vi "Load XML.vi"(8 "error in (no error)":errorcluster, 11 "path to XML document":path) -> (0 "error out":errorcluster, 3 "Map":map{string, T1}(c390))   [LabVIEW 2025]
uses:
  Controls/bd.ctl
  Classes/Node/Node.lvclass
  Controls/wire.ctl
  Controls/Terminal.ctl
  <vilib>/xml/Load XML File.vi
  <vilib>/xml/NI_XML.lvlib
  <vilib>/httpClient/LabVIEWHTTPClient.lvlib
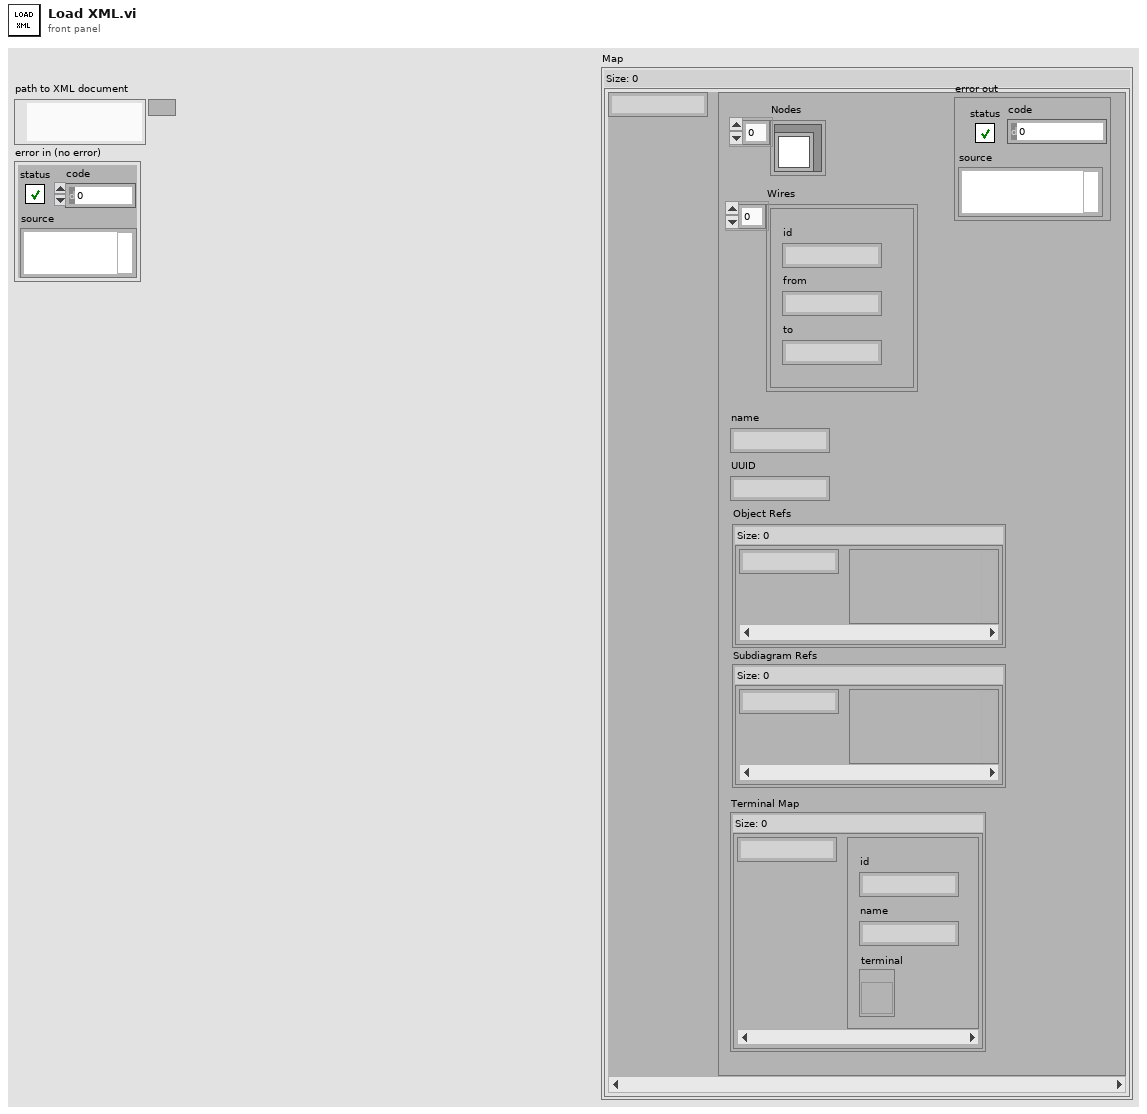
[diagram p1: front panel]
types:
  T1 = typedef "bd.ctl" = cluster{"Nodes":refnum<class "Node.lvclass">[], "Wires":T2[], "name":string, "UUID":string, "Object Refs":map{string, variant}, "Subdiagram Refs":map{string, variant}, "Terminal Map":map{string, T3}}
  T2 = typedef "wire.ctl" = cluster{"id":string, "from":string, "to":string}
  T3 = typedef "Terminal.ctl" = cluster{"id":string, "name":string, "terminal":refnum<vi>}
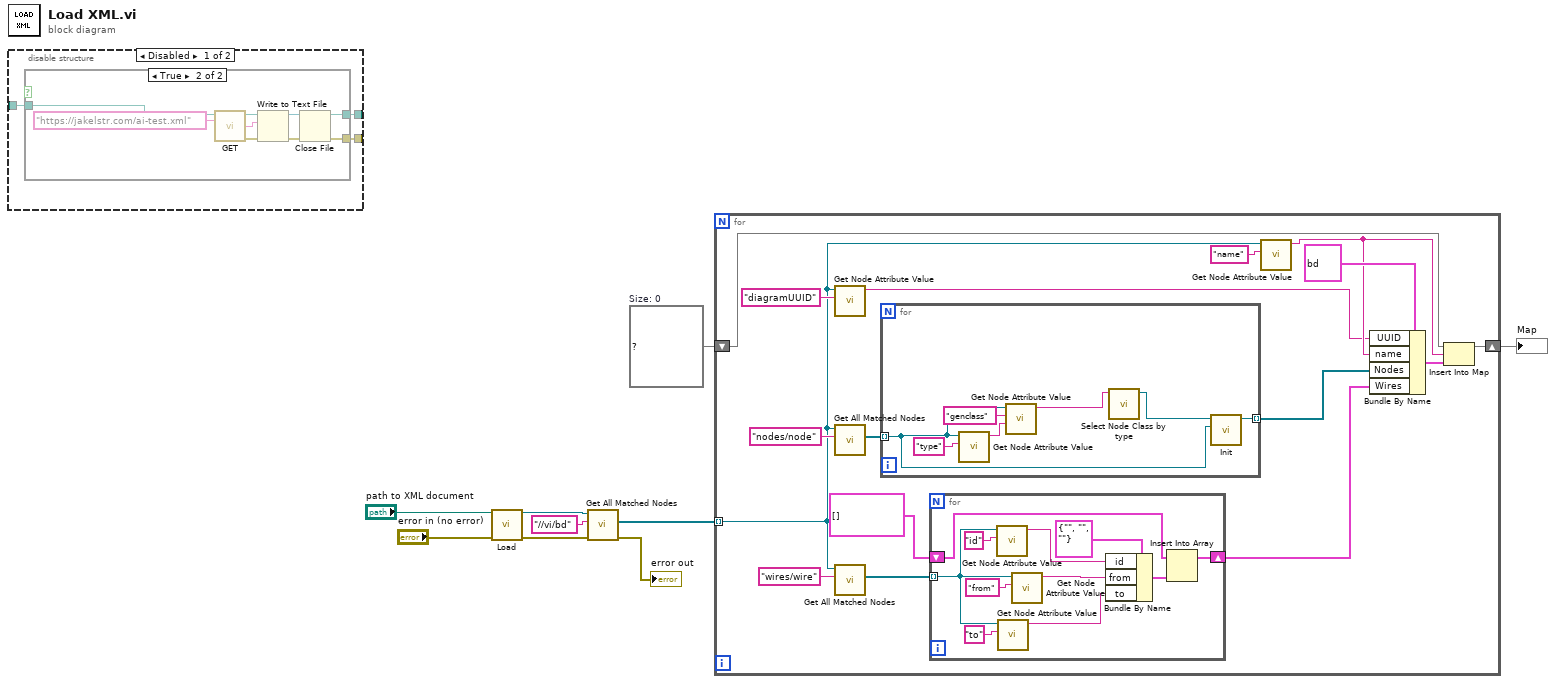
[diagram p0: block diagram]
diagram:
  w6 = map{string, T1} {}  # Size: 0
  n1 = disable-structure shown="Disabled" {
    disable-tunnel: [w12 _] -> _
    disable-tunnel: [w11 _] -> _
    disable-tunnel: _ -> [w10 _]
    frame Disabled {
      n2 = case shown="True" {
        selector: _ -> [_ _]
        tunnel: [_ w21] -> w12
        tunnel: [w13 w15] -> w11
        tunnel: w10 -> [w13 w14]
        frame False {
        }
        frame True {
          n3 = call <vilib>:"GET.vi"("url"="https://jakelstr.com/ai-test.xml") -> ("body"=w18:string, "error out"=w19:errorcluster)  [unwired: 11 in, 2 out]
          n4 = Write to Text File(file (use dialog)=w14, text=w18, error in=w19) -> (refnum out=w16:refnum<file>, error out=w17:errorcluster)  [unwired: 1 in, 1 out]
          n5 = Close File(refnum=w16, error in=w17) -> (path=w15:path, error out=w21:errorcluster)
        }
      }
    }
    frame Enabled {
    }
  }
  n6 = call-poly <vilib>:"Load.vi"("path to XML document"="path to XML document", "error in (no error)"="error in (no error)") -> ("DOM document out"=w8:refnum<k20>, "error out"=w9:errorcluster)  [unwired: 11 in, 1 out]
  n7 = call <vilib>:"Get All Matched Nodes.vi"("error in (no error)"=w9, "XPath expression"="//vi/bd", "node in"=w8) -> ("error out"=→"error out":errorcluster, "node result array"=w5:refnum<k20>[])  [unwired: 6 in, 1 out]
  n8 = for {
    tunnel: w5 -> [w22] mode=indexing
    shift-right: [w36] -> w4
    shift-left: w6 -> [w37]
    n9 = call "Get Node Attribute Value.vi"("Attribute Name"="diagramUUID", "Refnum in"=w22) -> ("Value"=w23:string)  [unwired: 9 in]
    n10 = call <vilib>:"Get All Matched Nodes.vi"("XPath expression"="nodes/node", "node in"=w22) -> ("node result array"=w31:refnum<k20>[])  [unwired: 7 in, 2 out]
    n11 = call <vilib>:"Get All Matched Nodes.vi"("XPath expression"="wires/wire", "node in"=w22) -> ("node result array"=w27:refnum<k20>[])  [unwired: 7 in, 2 out]
    n12 = for {
      tunnel: w31 -> [w51] mode=indexing
      tunnel: [w55] -> w30 mode=indexing
      n13 = call "Get Node Attribute Value.vi"("Attribute Name"="type", "Refnum in"=w51) -> ("Value"=w52:string)  [unwired: 9 in]
      n14 = call "Get Node Attribute Value.vi"("Default Value"=w52, "Attribute Name"="genclass", "Refnum in"=w51) -> ("Value"=w49:string)  [unwired: 8 in]
      n15 = call "Select Node Class by type.vi"("Value"=w49) -> ("Node out"=w53:refnum<class "Node.lvclass">)  [unwired: 10 in]
      n16 = call-dynamic "Init.vi"("Node Reg"=w51, "Node in"=w53) -> ("Node out"=w55:refnum<class "Node.lvclass">)  [unwired: 8 in, 1 out]
    }
    n17 = for {
      tunnel: w27 -> [w43] mode=indexing
      shift-right: [w47] -> w26
      shift-left: T2[] [] ("Wires") -> [w48]
      n18 = call "Get Node Attribute Value.vi"("Attribute Name"="id", "Refnum in"=w43) -> ("Value"=w41:string)  [unwired: 9 in]
      n19 = call "Get Node Attribute Value.vi"("Attribute Name"="to", "Refnum in"=w43) -> ("Value"=w39:string)  [unwired: 9 in]
      n20 = call "Get Node Attribute Value.vi"("Attribute Name"="from", "Refnum in"=w43) -> ("Value"=w40:string)  [unwired: 9 in]
      n21 = Bundle By Name(cluster=T2 {"id"="", "from"="", "to"=""} ("new element/subarray"), "id"=w41, "from"=w40, "to"=w39) -> (w38:T2)
      n22 = Insert Into Array(array=w48, new element=w38) -> (w47:T2[])  [unwired: 1 in]
    }
    n23 = call "Get Node Attribute Value.vi"("Attribute Name"="name", "Refnum in"=w22) -> ("Value"=w25:string)  [unwired: 9 in]
    n24 = Bundle By Name(cluster=T1 {"Nodes"=[], "Wires"=[], "name"="", "UUID"="", "Object Refs"={}, "Subdiagram Refs"={}, "Terminal Map"={}} ("Block Diagram"), "UUID"=w23, "name"=w25, "Nodes"=w30, "Wires"=w26) -> (w34:T1)
    n25 = Insert Into Map(map in=w37, key=w25, value=w34) -> (map out=w36:map{string, T1})  [unwired: 2 out]
  }
  "Map" <- w4
